vi "Meas Proc QWTB Update Result Table Variable Info.vi"(8 "error in":errorcluster, 11 "QWTB result session in":T1) -> (0 "error out":errorcluster)   [LabVIEW 2013]
doc: "This VI will take selection of the QWTB results table and finds description for the selected row in the QWTB result session. It will display it in the info indicator."
uses:
  Meas Proc QWTB Viewer References.ctl
  Meas Proc QWTB View Max Dim.ctl
  Meas Proc QWTB View Uncertainty Mode.ctl
  Meas Proc QWTB View Group Mode.ctl
  Meas Proc QWTB View Phase Mode.ctl
  varilib/SGUI Assign Multiple Strings With Tags By Label.vi
  varilib/varilib.lvlib
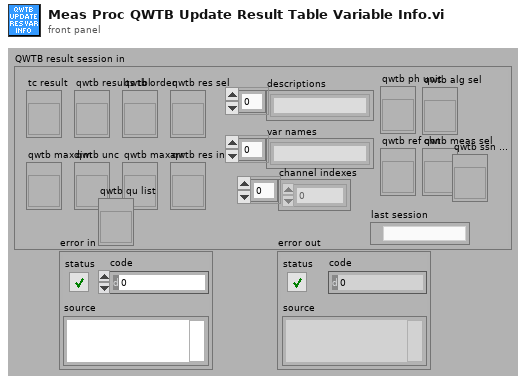
[diagram p1: front panel]
types:
  T1 = typedef "Meas Proc QWTB Viewer References.ctl" = cluster{"tc result":refnum<vi>, "qwtb results tbl":refnum<vi>, "qwtb maxdim":refnum<vi>, "qwtb unc":refnum<vi>, "qwtb order":refnum<vi>, "qwtb maxarr":refnum<vi>, "qwtb res sel":refnum<vi>, "qwtb res info":refnum<vi>, "descriptions":string[], "var names":string[], "channel indexes":i32[], "qwtb ref chn":refnum<vi>, "qwtb ph unit":refnum<vi>, "qwtb alg sel":refnum<vi>, "qwtb meas sel":refnum<vi>, "qwtb ssn info":refnum<vi>, "last session":path, "qwtb qu list":refnum<vi>}
  T2 = typedef "LVRowAndColumnTypeDef.ctl" = cluster{"Row":i32, "Column":i32}
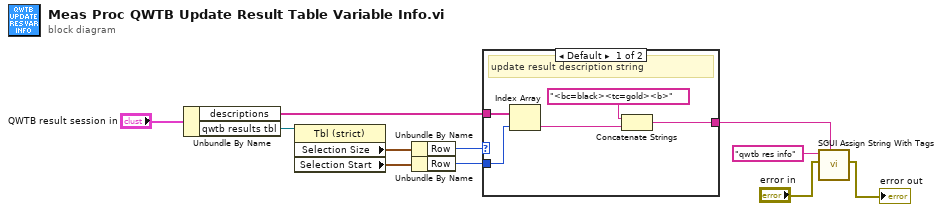
[diagram p0: block diagram]
diagram:
  n1 = Unbundle By Name("QWTB result session in") -> ("descriptions"=w11:string[], "qwtb results tbl"=w6:refnum<vi>)
  n2 = property class="Tbl (strict)"(reference=w6) -> ("Selection Size"=w7:T2, "Selection Start"=w9:T2)  [unwired: 1 in, 2 out]
  n3 = Unbundle By Name(w7) -> ("Row"=w8:i32)
  n4 = Unbundle By Name(w9) -> ("Row"=w10:i32)
  n5 = case shown="Default" w8 {
    tunnel: w10 -> [w15 _]
    tunnel: w11 -> [w16 _]
    tunnel: [w12 _] -> w3
    frame Default {
      # "update result description string"
      n6 = Index Array(array=w16, index=w15) -> (element=w13:string)
      n7 = Concatenate Strings("<bc=black><tc=gold><b>" ("string (empty)"), w13) -> (w12:string)
    }
    frame 0 {
    }
  }
  n8 = call-poly "SGUI Assign String With Tags.vi"("error in"="error in", "label(s) (empty)"="qwtb res info", "string (empty)"=w3) -> ("error out"=→"error out":errorcluster)  [unwired: 7 in, 1 out]
